vi "clear Session Data.vi"(0 "Session in":refnum<class "Remote Connection Session.lvclass">, 11 "error in":errorcluster) -> (4 "Session out":refnum<class "Remote Connection Session.lvclass">, 15 "error out":errorcluster)   [LabVIEW 2012, in "REx.lvlib" / "Remote Connection Session.lvclass"]
uses:
  Remote Connection Session.lvclass
  <userlib>/_Session Fwk/Session - Root.lvclass
  Remote Connection Session.lvclass/Remote Connection Session.ctl
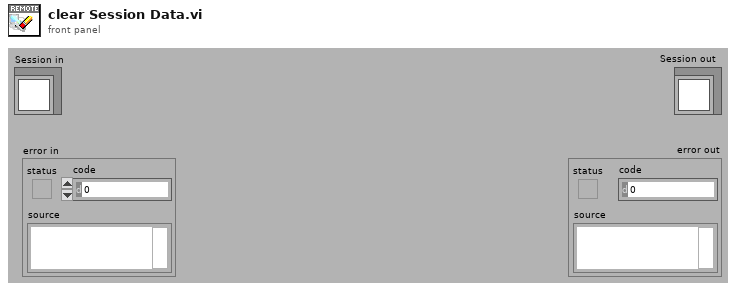
[diagram p1: front panel]
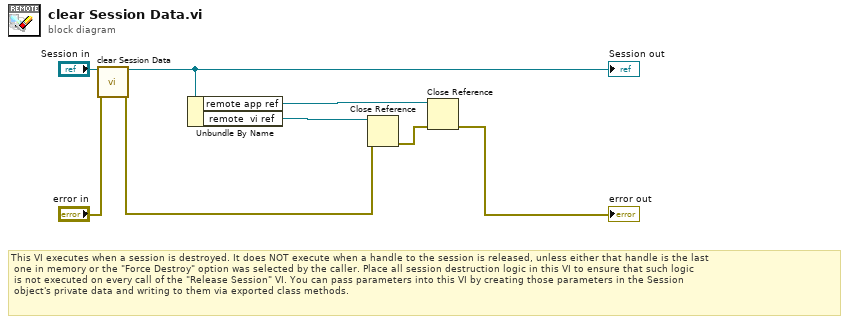
[diagram p0: block diagram]
diagram:
  # "This VI executes when a session is destroyed. It does NOT execute when a handle to the session is released, unless either that handle is the last\n one in memory or the \"Force Destroy\" option was selected by the caller. Place all session destruction logic in this VI to ensure that such logic\n is not executed on every call of the \"Release Session\" VI. You can pass parameters into this VI by creating those parameters in the Session \n object's private data and writing to them via exported class methods."
  n1 = call-parent "clear Session Data.vi"("OBJ - Measurement Session in"="Session in", "error in"="error in") -> ("OBJ - Measurement Session out"=w4:refnum<class "Remote Connection Session.lvclass">, "error out"=w5:errorcluster)  [unwired: 12 in]
  "Session out" <- w4
  n2 = Unbundle By Name(w4) -> ("remote app ref"=w2:refnum<vi>, "remote  vi ref"=w6:refnum<vi>)
  n3 = Close Reference(reference=w6, error in (no error)=w5) -> (error out=w3:errorcluster)
  n4 = Close Reference(reference=w2, error in (no error)=w3) -> (error out=→"error out":errorcluster)
